vi "SetFormatter.vi"(8 "error in (no error)":errorcluster, 9 "Formatter in":refnum<class "Formatter.lvclass">, 10 "Handler in":refnum<class "Handler.lvclass">, 11 "Logger in":refnum<class "Logger.lvclass">) -> (0 "error out":errorcluster, 1 "Formatter out":refnum<class "Formatter.lvclass">, 2 "Handler out":refnum<class "Handler.lvclass">, 3 "Logger out":refnum<class "Logger.lvclass">)   [LabVIEW 2022 SP3, in "Logger.lvlib" / "Logger.lvclass"]
uses:
  Logger.lvclass
  Logger.lvclass/Logger.ctl
  Formatter/Formatter.lvclass
  Handler/Handler.lvclass
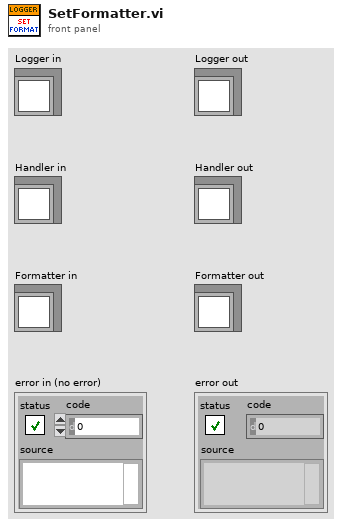
[diagram p1: front panel]
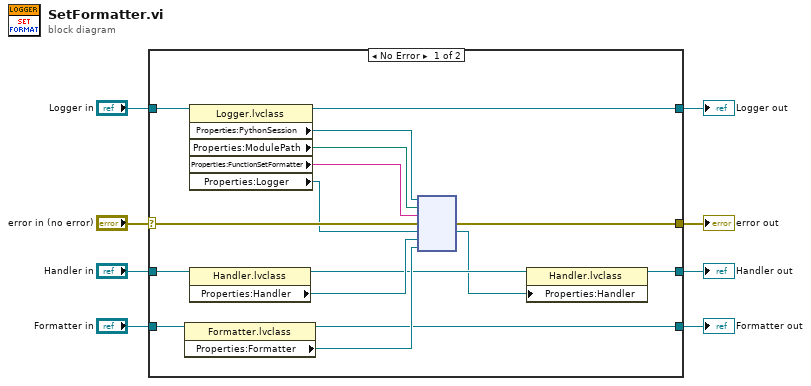
[diagram p0: block diagram]
diagram:
  n1 = case shown="No Error" "error in (no error)" {
    selector: "error in (no error)" -> [w22 w26]
    tunnel: [w21 w26] -> w6
    tunnel: [w23 w25] -> w5
    tunnel: "Logger in" -> [w24 w25]
    tunnel: "Handler in" -> [w16 _]
    tunnel: "Formatter in" -> [w14 _]
    tunnel: [w10 _] -> w2
    tunnel: [w9 _] -> w1
    frame No Error {
      n2 = property class="Formatter.lvclass"(reference=w14) -> (reference out=w9:refnum<class "Formatter.lvclass">, "Properties:Formatter"=w13:refnum<k38>)  [unwired: 1 in, 1 out]
      n3 = property class="Logger.lvclass"(reference=w24) -> (reference out=w23:refnum<class "Logger.lvclass">, "Properties:PythonSession"=w20:refnum<k35>, "Properties:ModulePath"=w18:path, "Properties:FunctionSetFormatter"=w19:string, "Properties:Logger"=w17:refnum<k38>)  [unwired: 1 in, 1 out]
      n4 = property class="Handler.lvclass"(reference=w16) -> (reference out=w12:refnum<class "Handler.lvclass">, "Properties:Handler"=w15:refnum<k38>)  [unwired: 1 in, 1 out]
      n5 = node(w20, w18, w19, w22, w17, w15, w13) -> (w21:errorcluster, w11:refnum<k38>)  [unwired: 2 in, 3 out]
      n6 = property class="Handler.lvclass"(reference=w12, "Properties:Handler"=w11) -> (reference out=w10:refnum<class "Handler.lvclass">)  [unwired: 1 in, 1 out]
    }
    frame Error {
    }
  }
  "error out" <- w6
  "Logger out" <- w5
  "Handler out" <- w2
  "Formatter out" <- w1
